vi "Attributes Metadata.vi"(7 "Actor in":refnum<class "Actor.lvclass">) -> (2 "Attributes Metadata":refnum<class "Attributes Metadata.lvclass">)   [LabVIEW 2020, in "jettl.lvlib" / "Read Parent Attributes.lvlib"]
uses:
  Read Parent Attributes.lvlib
  Actor/Actor.lvclass
  Attributes Metadata/Attributes Metadata.lvclass
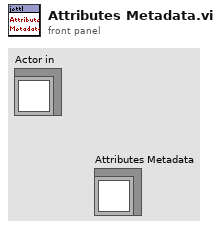
[diagram p1: front panel]
types:
  T1 = typedef "jettl.lvlib/Attributes.ctl" = cluster{"Unified Msgs":T2, "Unified Leaf":bool, "Edge Actors":refnum<class "Actor.lvclass">[], "Core Actors":refnum<class "Actor.lvclass">[], "Root":bool, "Alias":string, "UID":i32, "Transport":refnum<class "Transport.lvclass">, "This VI":refnum<vi>, "Attributes Metadata":refnum<class "Attributes Metadata.lvclass">, "Post-Setup Actors":refnum<class "Actor.lvclass">[]}
  T2 = typedef "jettl.lvlib/Msgs.ctl" = set{refnum<class "Msg.lvclass">}
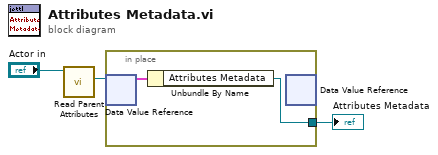
[diagram p0: block diagram]
diagram:
  n1 = call-dynamic "Read Parent Attributes.vi"("Actor in"="Actor in") -> ("Parent Attributes"=w2:refnum<data-value>)  [unwired: 10 in]
  n2 = in-place {
    in-place-border: [w4] -> w1
    n3 = in-place-dvr #1(w2) -> (w5:T1)  [unwired: 1 out]
    n4 = Unbundle By Name(w5) -> ("Attributes Metadata"=w4:refnum<class "Attributes Metadata.lvclass">)
    n5 = in-place-dvr #1() -> ()  [unwired: 1 in, 2 out]
  }
  "Attributes Metadata" <- w1
